vi "7.8-TCP Data Server.vi"() -> ()   [LabVIEW 2011]
doc: "Sends a specified waveform through a TCP port. The VI first listens for a connection and, once established, sends the number of bytes to be sent followed by the data. After the data is sent, the VI waits for an 'all received' signal from the client and then breaks the connection.\n\n<B>Note:</B> Requires the Data Client.vi located in the same library as this VI."
uses:
  7.0-Global.vi
panel:
  in  "Port":u16=22234 min=1025 step=1
  # "Instructions:\n1. Open the Data Client.vi\n2. Run This VI first.\n3. Run the Data Client.vi Second.\n4. Adjust the # of Points Function, and Noise Level controls.\n5. Observe the Chart on the Data Client.vi.\n6. Stop This VI. The Data Client.vi will time out and stop."
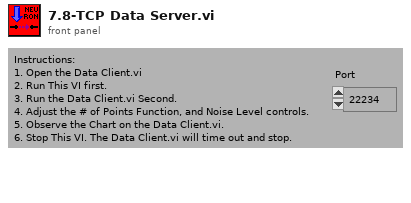
[diagram p1: front panel]
types:
  T1 = typedef "6.0-OCU to Forebrain Neuron.ctl" = cluster{"6.1 Act":T2, "7.6 - GPS Waypoints Data":T4}
  T2 = typedef "6.1-Act.ctl" = cluster{"6.1-Saitek Controller":T3, "Joystick Mode":bool, "Shutdown":bool, "Reset":bool, "Begin":bool}
  T3 = typedef "6.1-UDP Saitek.ctl" = cluster{"Stop":bool, "Setpoint":bool, "Run":bool, "Restart":bool, "Shutdown":bool, "Joystick\nMode 1":bool, "Joystick\nMode 2":bool, "Joystick \nMode 3":bool, "Joystick Mode 4":bool, "10":bool, "11":bool, "Pitch":sgl, "Roll":sgl, "Yaw":sgl, "Left":sgl, "Right":sgl}
  T4 = typedef "7.6 - GPS Waypoint Def.ctl" = cluster{"GPS Waypoint Center (Lat, Long)":dbl[], "5.1.1 MDF GPS":T5}
  T5 = typedef "MDF Array LatLong.ctl" = T6[]
  T6 = typedef "MDF LatLong.ctl" = cluster{"Waypoint #":dbl, "Latitude (waypoint)":ext, "Longitude  (waypoint)":ext}
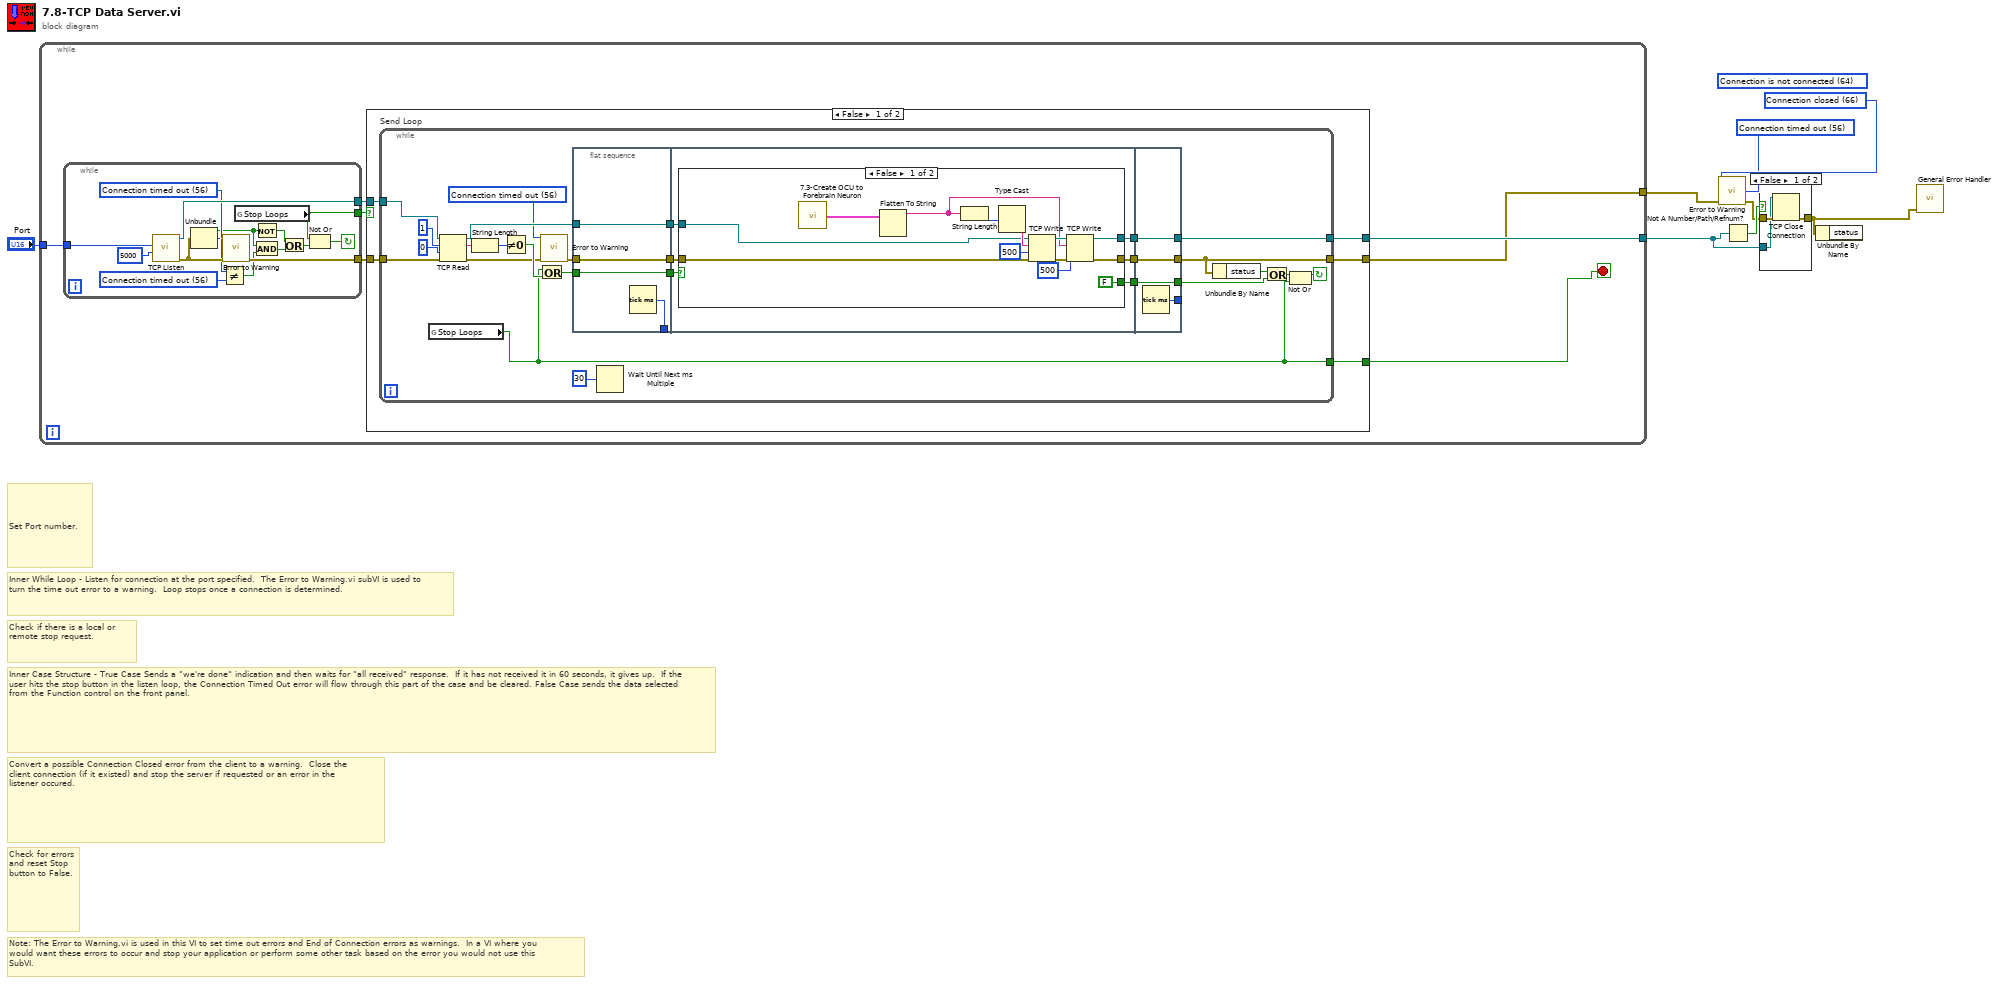
[diagram p0: block diagram]
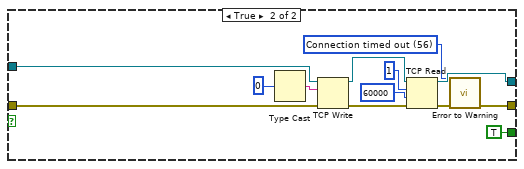
[diagram p3: hidden frame]
diagram:
  w3 = 56 items=["No Error", "Argument Error", "Memory Full", "Out of Zone", "End of File", "File Already Open", "Generic File IO Error", "File Not Found", "File Permission Error", "Disk Full", "Duplicate Path", "Too Many Files Open", "Not Enabled", "Resource File Not Found", "Cannot Add Resource", "Resource Not Found", "Image Not Found", "Image Memory Error", "Pen Does Not Exist", "Config Bad Type", "Config Token Not Found", "Config Parse Error", "Config Memory Error", "Bad External Code Format", "Bad External Code Offset", "External Code Not Present", "Null Window", "Destroy Window Mixup", "Null Menu", "Print Aborted", "Bad Print Record", "Print Driver Error", "Windows Error During Print", "Memory Error During Print", "Print Dialog Error", "Generic Print Error", "Invalid Device Refnum", "Device Not Found", "Device Parameter Error", "Device Unit Error", "Can't Open Device", "Device Call Aborted", "Generic Error", "Cancelled By User", "Object ID Too Low", "Object ID Too High", "Object Not In Heap", "Unknown Heap", "Bad DefProc ID", "DefProc Not In Table", "Message Out Of Range", "Null Method", "Unknown Message", "Manager Call Not Supported", "Bad address", "Connection In progress", "Connection timed out", "Connection is already in progress", "Network attribute not supported", "Network error", "Address in use", "System out of memory", "Connection aborted", "Connection refused", "Connection is not connected", "Connection is already connected", "Connection closed", "Initialize error (interapplication manager)", "Bad occurrence", "Wait on unbound occurrence handler", "Occurrence queue overflow", "Bad path", "Semaphore not signaled", "Unrecognized type (interapplication manager)"] ("3rd Error to Convert")
  w5 = 66 items=["No Error", "Argument Error", "Memory Full", "Out of Zone", "End of File", "File Already Open", "Generic File IO Error", "File Not Found", "File Permission Error", "Disk Full", "Duplicate Path", "Too Many Files Open", "Not Enabled", "Resource File Not Found", "Cannot Add Resource", "Resource Not Found", "Image Not Found", "Image Memory Error", "Pen Does Not Exist", "Config Bad Type", "Config Token Not Found", "Config Parse Error", "Config Memory Error", "Bad External Code Format", "Bad External Code Offset", "External Code Not Present", "Null Window", "Destroy Window Mixup", "Null Menu", "Print Aborted", "Bad Print Record", "Print Driver Error", "Windows Error During Print", "Memory Error During Print", "Print Dialog Error", "Generic Print Error", "Invalid Device Refnum", "Device Not Found", "Device Parameter Error", "Device Unit Error", "Can't Open Device", "Device Call Aborted", "Generic Error", "Cancelled By User", "Object ID Too Low", "Object ID Too High", "Object Not In Heap", "Unknown Heap", "Bad DefProc ID", "DefProc Not In Table", "Message Out Of Range", "Null Method", "Unknown Message", "Manager Call Not Supported", "Bad address", "Connection In progress", "Connection timed out", "Connection is already in progress", "Network attribute not supported", "Network error", "Address in use", "System out of memory", "Connection aborted", "Connection refused", "Connection is not connected", "Connection is already connected", "Connection closed", "Initialize error (interapplication manager)", "Bad occurrence", "Wait on unbound occurrence handler", "Occurrence queue overflow", "Bad path", "Semaphore not signaled", "Unrecognized type (interapplication manager)"] ("2nd Error to Convert")
  (unwired) 64 items=["No Error", "Argument Error", "Memory Full", "Out of Zone", "End of File", "File Already Open", "Generic File IO Error", "File Not Found", "File Permission Error", "Disk Full", "Duplicate Path", "Too Many Files Open", "Not Enabled", "Resource File Not Found", "Cannot Add Resource", "Resource Not Found", "Image Not Found", "Image Memory Error", "Pen Does Not Exist", "Config Bad Type", "Config Token Not Found", "Config Parse Error", "Config Memory Error", "Bad External Code Format", "Bad External Code Offset", "External Code Not Present", "Null Window", "Destroy Window Mixup", "Null Menu", "Print Aborted", "Bad Print Record", "Print Driver Error", "Windows Error During Print", "Memory Error During Print", "Print Dialog Error", "Generic Print Error", "Invalid Device Refnum", "Device Not Found", "Device Parameter Error", "Device Unit Error", "Can't Open Device", "Device Call Aborted", "Generic Error", "Cancelled By User", "Object ID Too Low", "Object ID Too High", "Object Not In Heap", "Unknown Heap", "Bad DefProc ID", "DefProc Not In Table", "Message Out Of Range", "Null Method", "Unknown Message", "Manager Call Not Supported", "Bad address", "Connection In progress", "Connection timed out", "Connection is already in progress", "Network attribute not supported", "Network error", "Address in use", "System out of memory", "Connection aborted", "Connection refused", "Connection is not connected", "Connection is already connected", "Connection closed", "Initialize error (interapplication manager)", "Bad occurrence", "Wait on unbound occurrence handler", "Occurrence queue overflow", "Bad path", "Semaphore not signaled", "Unrecognized type (interapplication manager)"] ("1st Error to Convert")
  # "Check for errors\nand reset Stop \nbutton to False."
  # "Inner Case Structure - True Case Sends a \"we're done\" indication and then waits for \"all received\" response.  If it has not received it in 60 seconds, it gives up.  If the user hits the stop button in the listen loop, the Connection Timed Out error will flow through this part of the case and be cleared. False Case sends the data selected from the Function control on the front panel."
  # "Check if there is a local or remote stop request."
  # "Set Port number."
  # "Inner While Loop - Listen for connection at the port specified.  The Error to Warning.vi subVI is used to turn the time out error to a warning.  Loop stops once a connection is determined."
  # "Note: The Error to Warning.vi is used in this VI to set time out errors and End of Connection errors as warnings.  In a VI where you would want these errors to occur and stop your application or perform some other task based on the error you would not use this SubVI."
  # "Convert a possible Connection Closed error from the client to a warning.  Close the client connection (if it existed) and stop the server if requested or an error in the listener occured."
  n1 = while {
    tunnel: "Port" -> [w15]
    tunnel: [w10] -> w2
    tunnel: [w9] -> w1
    stop <- w11 stop-if-true
    n2 = while {
      tunnel: [w16] -> w12
      tunnel: [w25] -> w13
      tunnel: [w29] -> w14
      tunnel: w15 -> [w30]
      stop <- w27 continue-if-true
      w23 = 56 items=["No Error", "Argument Error", "Memory Full", "Out of Zone", "End of File", "File Already Open", "Generic File IO Error", "File Not Found", "File Permission Error", "Disk Full", "Duplicate Path", "Too Many Files Open", "Not Enabled", "Resource File Not Found", "Cannot Add Resource", "Resource Not Found", "Image Not Found", "Image Memory Error", "Pen Does Not Exist", "Config Bad Type", "Config Token Not Found", "Config Parse Error", "Config Memory Error", "Bad External Code Format", "Bad External Code Offset", "External Code Not Present", "Null Window", "Destroy Window Mixup", "Null Menu", "Print Aborted", "Bad Print Record", "Print Driver Error", "Windows Error During Print", "Memory Error During Print", "Print Dialog Error", "Generic Print Error", "Invalid Device Refnum", "Device Not Found", "Device Parameter Error", "Device Unit Error", "Can't Open Device", "Device Call Aborted", "Generic Error", "Cancelled By User", "Object ID Too Low", "Object ID Too High", "Object Not In Heap", "Unknown Heap", "Bad DefProc ID", "DefProc Not In Table", "Message Out Of Range", "Null Method", "Unknown Message", "Manager Call Not Supported", "Bad address", "Connection In progress", "Connection timed out", "Connection is already in progress", "Network attribute not supported", "Network error", "Address in use", "System out of memory", "Connection aborted", "Connection refused", "Connection is not connected", "Connection is already connected", "Connection closed", "Initialize error (interapplication manager)", "Bad occurrence", "Wait on unbound occurrence handler", "Occurrence queue overflow", "Bad path", "Semaphore not signaled", "Unrecognized type (interapplication manager)"] ("1st Error to Convert")
      w24 = 56 items=["No Error", "Argument Error", "Memory Full", "Out of Zone", "End of File", "File Already Open", "Generic File IO Error", "File Not Found", "File Permission Error", "Disk Full", "Duplicate Path", "Too Many Files Open", "Not Enabled", "Resource File Not Found", "Cannot Add Resource", "Resource Not Found", "Image Not Found", "Image Memory Error", "Pen Does Not Exist", "Config Bad Type", "Config Token Not Found", "Config Parse Error", "Config Memory Error", "Bad External Code Format", "Bad External Code Offset", "External Code Not Present", "Null Window", "Destroy Window Mixup", "Null Menu", "Print Aborted", "Bad Print Record", "Print Driver Error", "Windows Error During Print", "Memory Error During Print", "Print Dialog Error", "Generic Print Error", "Invalid Device Refnum", "Device Not Found", "Device Parameter Error", "Device Unit Error", "Can't Open Device", "Device Call Aborted", "Generic Error", "Cancelled By User", "Object ID Too Low", "Object ID Too High", "Object Not In Heap", "Unknown Heap", "Bad DefProc ID", "DefProc Not In Table", "Message Out Of Range", "Null Method", "Unknown Message", "Manager Call Not Supported", "Bad address", "Connection In progress", "Connection timed out", "Connection is already in progress", "Network attribute not supported", "Network error", "Address in use", "System out of memory", "Connection aborted", "Connection refused", "Connection is not connected", "Connection is already connected", "Connection closed", "Initialize error (interapplication manager)", "Bad occurrence", "Wait on unbound occurrence handler", "Occurrence queue overflow", "Bad path", "Semaphore not signaled", "Unrecognized type (interapplication manager)"] ("1st Error to Convert")
      n3 = call <vilib>:"TCP Listen.vi"("timeout ms (wait forever: -1)"=5000, "port"=w30) -> ("error out"=w26:errorcluster, "connection ID"=w29:refnum<k5>)  [unwired: 5 in, 3 out]
      n4 = Unbundle(w26) -> ("status"=w21:bool, "code"=w22:i32)  [unwired: 1 out]
      n5 = Not Equal?(x=w22, y=w23) -> (x != y?=w20:bool)
      n6 = call <vilib>:"Error to Warning.vi"("1st Error to Convert"=w24, "error in"=w26) -> ("warning out"=w25:errorcluster)  [unwired: 13 in]
      n7 = global read "7.0-Global.vi" "Stop Loops"() -> (w16:bool)
      n8 = Not(x=w21) -> (.not. x?=w19:bool)
      n9 = And(x=w21, y=w20) -> (x .and. y?=w18:bool)
      n10 = Or(x=w19, y=w18) -> (x .or. y?=w17:bool)
      n11 = Not Or(1:w17, 2:w16) -> (0:w27:bool)
    }
    n12 = case shown="False" w12 {
      selector: w12 -> [_ w102]
      tunnel: [w31 w103] -> w9
      tunnel: w14 -> [w33 w104]
      tunnel: w13 -> [w32 w103]
      tunnel: [w35 w104] -> w10
      tunnel: [w34 w102] -> w11
      frame False {
        n13 = while "Send Loop" {
          tunnel: [w36] -> w34
          tunnel: w32 -> [w58]
          tunnel: [w49] -> w31
          tunnel: [w54] -> w35
          tunnel: w33 -> [w57]
          stop <- w37 continue-if-true
          w47 = 56 items=["No Error", "Argument Error", "Memory Full", "Out of Zone", "End of File", "File Already Open", "Generic File IO Error", "File Not Found", "File Permission Error", "Disk Full", "Duplicate Path", "Too Many Files Open", "Not Enabled", "Resource File Not Found", "Cannot Add Resource", "Resource Not Found", "Image Not Found", "Image Memory Error", "Pen Does Not Exist", "Config Bad Type", "Config Token Not Found", "Config Parse Error", "Config Memory Error", "Bad External Code Format", "Bad External Code Offset", "External Code Not Present", "Null Window", "Destroy Window Mixup", "Null Menu", "Print Aborted", "Bad Print Record", "Print Driver Error", "Windows Error During Print", "Memory Error During Print", "Print Dialog Error", "Generic Print Error", "Invalid Device Refnum", "Device Not Found", "Device Parameter Error", "Device Unit Error", "Can't Open Device", "Device Call Aborted", "Generic Error", "Cancelled By User", "Object ID Too Low", "Object ID Too High", "Object Not In Heap", "Unknown Heap", "Bad DefProc ID", "DefProc Not In Table", "Message Out Of Range", "Null Method", "Unknown Message", "Manager Call Not Supported", "Bad address", "Connection In progress", "Connection timed out", "Connection is already in progress", "Network attribute not supported", "Network error", "Address in use", "System out of memory", "Connection aborted", "Connection refused", "Connection is not connected", "Connection is already connected", "Connection closed", "Initialize error (interapplication manager)", "Bad occurrence", "Wait on unbound occurrence handler", "Occurrence queue overflow", "Bad path", "Semaphore not signaled", "Unrecognized type (interapplication manager)"] ("1st Error to Convert")
          n14 = global read "7.0-Global.vi" "Stop Loops"() -> (w36:bool)
          n15 = TCP Read(connection ID=w57, bytes to read=1, error in (no error)=w58, 9:0) -> (connection ID out=w55:refnum<k5>, data out=w56:string, error out=w46:errorcluster)  [unwired: 1 in]
          n16 = String Length(string=w56) -> (length=w52:i32)
          n17 = Not Equal To 0?(x=w52) -> (x != 0?=w51:bool)
          n18 = Or(x=w36, y=w51) -> (x .or. y?=w50:bool)
          n19 = call <vilib>:"Error to Warning.vi"("1st Error to Convert"=w47, "error in"=w46) -> ("warning out"=w45:errorcluster)  [unwired: 13 in]
          n20 = flat-sequence {
            tunnel: w45 -> [w63]
            tunnel: w50 -> [w64]
            tunnel: w55 -> [w65]
            tunnel: [w65] -> w41
            tunnel: [w64] -> w40
            tunnel: [w63] -> w39
            tunnel: [w62] -> _
            tunnel: [w70] -> w44
            tunnel: [w69] -> w43
            tunnel: [w67] -> w42
            tunnel: w41 -> [w71]
            tunnel: w40 -> [w68]
            tunnel: w39 -> [w66]
            tunnel: [w99] -> w49
            tunnel: [w100] -> w53
            tunnel: [w101] -> w54
            tunnel: w44 -> [w101]
            tunnel: w43 -> [w100]
            tunnel: w42 -> [w99]
            tunnel: [w98] -> _
            frame #0 {
              n21 = Tick Count (ms)() -> (millisecond timer value=w62:u32)
            }
            frame #1 {
              n22 = case shown="False" w68 {
                tunnel: w66 -> [w76 w93]
                tunnel: w71 -> [w75 w91]
                tunnel: [w79 w95] -> w70
                tunnel: [w78 w86] -> w67
                tunnel: [FALSE TRUE] -> w69
                frame False {
                  n23 = call "7.3-Create OCU to Forebrain Neuron.vi"() -> ("output cluster"=w72:T1)
                  n24 = Flatten To String(anything=w72) -> (data string=w77:string)  [unwired: 3 in, 2 out]
                  n25 = String Length(string=w77) -> (length=w83:i32)
                  n26 = Type Cast(x=w83) -> (*(type *) &x=w82:string)  [unwired: 1 in]
                  n27 = TCP Write(connection ID=w75, data in=w82, error in (no error)=w76, 9:500 ("timeout ms (25000)")) -> (connection ID out=w80:refnum<k5>, error out=w81:errorcluster)  [unwired: 1 out]
                  n28 = TCP Write(connection ID=w80, data in=w77, error in (no error)=w81, 9:500 ("timeout ms (25000)")) -> (connection ID out=w79:refnum<k5>, error out=w78:errorcluster)  [unwired: 1 out]
                }
                frame True {
                  w85 = 56 items=["No Error", "Argument Error", "Memory Full", "Out of Zone", "End of File", "File Already Open", "Generic File IO Error", "File Not Found", "File Permission Error", "Disk Full", "Duplicate Path", "Too Many Files Open", "Not Enabled", "Resource File Not Found", "Cannot Add Resource", "Resource Not Found", "Image Not Found", "Image Memory Error", "Pen Does Not Exist", "Config Bad Type", "Config Token Not Found", "Config Parse Error", "Config Memory Error", "Bad External Code Format", "Bad External Code Offset", "External Code Not Present", "Null Window", "Destroy Window Mixup", "Null Menu", "Print Aborted", "Bad Print Record", "Print Driver Error", "Windows Error During Print", "Memory Error During Print", "Print Dialog Error", "Generic Print Error", "Invalid Device Refnum", "Device Not Found", "Device Parameter Error", "Device Unit Error", "Can't Open Device", "Device Call Aborted", "Generic Error", "Cancelled By User", "Object ID Too Low", "Object ID Too High", "Object Not In Heap", "Unknown Heap", "Bad DefProc ID", "DefProc Not In Table", "Message Out Of Range", "Null Method", "Unknown Message", "Manager Call Not Supported", "Bad address", "Connection In progress", "Connection timed out", "Connection is already in progress", "Network attribute not supported", "Network error", "Address in use", "System out of memory", "Connection aborted", "Connection refused", "Connection is not connected", "Connection is already connected", "Connection closed", "Initialize error (interapplication manager)", "Bad occurrence", "Wait on unbound occurrence handler", "Occurrence queue overflow", "Bad path", "Semaphore not signaled", "Unrecognized type (interapplication manager)"] ("1st Error to Convert")
                  n29 = Type Cast(x=0) -> (*(type *) &x=w88:string)  [unwired: 1 in]
                  n30 = TCP Write(connection ID=w91, data in=w88, error in (no error)=w93) -> (connection ID out=w90:refnum<k5>, error out=w92:errorcluster)  [unwired: 1 in, 1 out]
                  n31 = TCP Read(connection ID=w90, bytes to read=1, error in (no error)=w92, 9:60000) -> (connection ID out=w95:refnum<k5>, error out=w87:errorcluster)  [unwired: 1 in, 1 out]
                  n32 = call <vilib>:"Error to Warning.vi"("1st Error to Convert"=w85, "error in"=w87) -> ("warning out"=w86:errorcluster)  [unwired: 13 in]
                }
              }
            }
            frame #2 {
              n33 = Tick Count (ms)() -> (millisecond timer value=w98:u32)
            }
          }
          n34 = Wait Until Next ms Multiple(millisecond multiple=u32 30 ("milliseconds to wait")) -> ()  [unwired: 1 out]
          n35 = Unbundle By Name(w49) -> ("status"=w48:bool)
          n36 = Or(x=w48, y=w53) -> (x .or. y?=w61:bool)
          n37 = Not Or(1:w36, 2:w61) -> (0:w37:bool)
        }
      }
      frame True {
      }
    }
  }
  n38 = call <vilib>:"Error to Warning.vi"("2nd Error to Convert"=w5, "3rd Error to Convert"=w3, "error in"=w1) -> ("warning out"=w4:errorcluster)  [unwired: 12 in]
  n39 = Not A Number/Path/Refnum?(number/path/refnum=w2) -> (NaN/Path/Refnum?=w6:bool)
  n40 = case shown="False" w6 {
    tunnel: w4 -> [w107 w108]
    tunnel: w2 -> [w106 _]
    tunnel: [w105 w108] -> w7
    frame False {
      n41 = TCP Close Connection(connection ID=w106, error in (no error)=w107) -> (error out=w105:errorcluster)  [unwired: 1 in, 1 out]
    }
    frame True {
    }
  }
  n42 = Unbundle By Name(w7) -> ()  [unwired: 1 out]
  n43 = call <vilib>:"General Error Handler.vi"("error in (no error)"=w7) -> ()  [unwired: 10 in, 5 out]
